vi "Actor Core.vi"(8 "error in":cluster{"状态":bool, "代码":i32, "源":string} caption="错误输入", 11 "我的应用程序":refnum<class "多对一.lvclass">) -> (0 "error out":cluster{"状态":bool, "代码":i32, "源":string} caption="错误输出", 3 "操作者输出":refnum<class "Actor.lvclass">)   [LabVIEW 2015, in "多对一.lvlib" / "多对一.lvclass"]
doc: "Actor Core.vi包含操作者的主要消息处理循环。操作者通常位于该循环中，在各种消息到达时对消息进行处理。如Do.vi消息返回任何错误，该循环将停止运行，错误代码43将被作为“无错误停止”的标准信号发送给调用方。如需更改上述行为，可在子孙类的Handle Error.vi中对该部分逻辑进行重写。"
uses:
  <vilib>/ActorFramework/Actor/Actor.lvclass
  <vilib>/ActorFramework/Stop Msg/Stop Msg.lvclass
panel:
  in  "停止信号":bool
  out "事件记录":string
  in  "停止":bool
  in  "至客户端的消息":bool
  in  "至硬件的消息":bool
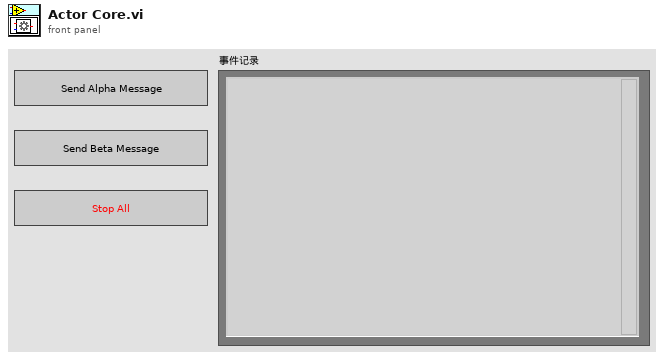
[diagram p1: front panel]
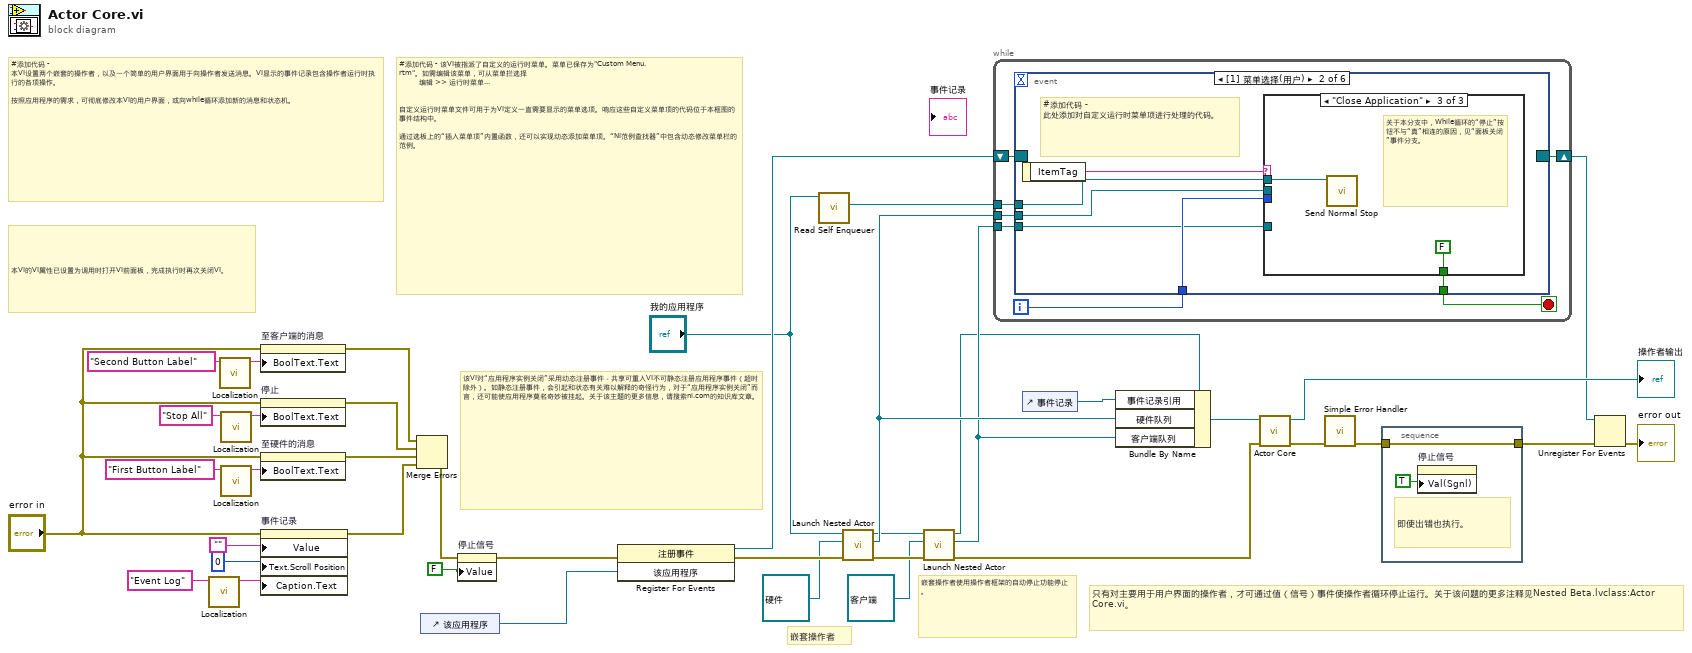
[diagram p0: block diagram]
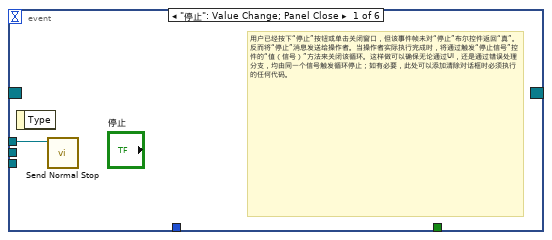
[diagram p2: hidden frame]
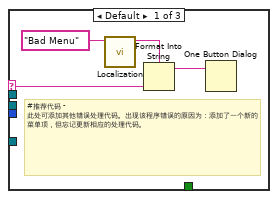
[diagram p3: hidden frame]
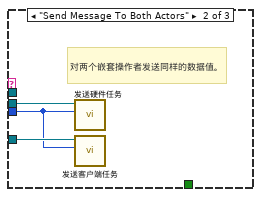
[diagram p4: hidden frame]
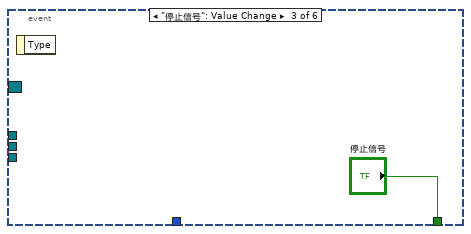
[diagram p5: hidden frame]
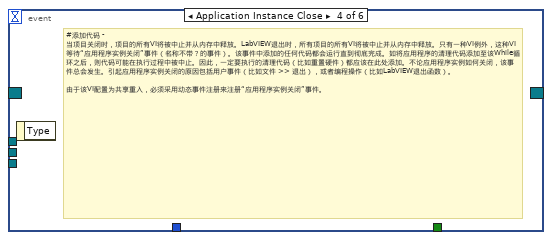
[diagram p6: hidden frame]
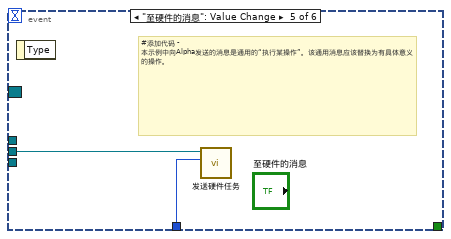
[diagram p7: hidden frame]
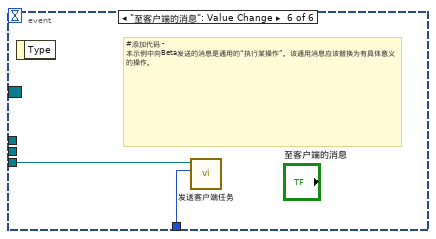
[diagram p8: hidden frame]
diagram:
  # "嵌套操作者"
  # "嵌套操作者使用操作者框架的自动停止功能停止。"
  # "#添加代码 - 该VI被指派了自定义的运行时菜单。菜单已保存为\"Custom Menu.rtm\"。如需编辑该菜单，可从菜单拦选择\n          编辑 >> 运行时菜单...\n\n\n自定义运行时菜单文件可用于为VI定义一直需要显示的菜单选项。响应这些自定义菜单项的代码位于本框图的事件结构中。\n\n通过选板上的“插入菜单项”内置函数，还可以实现动态添加菜单项。“NI范例查找器”中包含动态修改菜单栏的范例。"
  # "该VI对“应用程序实例关闭”采用动态注册事件－共享可重入VI不可静态注册应用程序事件（超时除外）。如静态注册事件，会引起和状态有关难以解释的奇怪行为，对于“应用程序实例关闭”而言，还可能使应用程序莫名奇妙被挂起。关于该主题的更多信息，请搜索ni.com的知识库文章。"
  # "本VI的VI属性已设置为调用时打开VI前面板，完成执行时再次关闭VI。"
  # "只有对主要用于用户界面的操作者，才可通过值（信号）事件使操作者循环停止运行。关于该问题的更多注释见Nested Beta.lvclass:Actor Core.vi。"
  # "#添加代码 - 本VI设置两个嵌套的操作者，以及一个简单的用户界面用于向操作者发送消息。VI显示的事件记录包含操作者运行时执行的各项操作。\n\n按照应用程序的需求，可彻底修改本VI的用户界面，或向while循环添加新的消息和状态机。"
  n1 = call "Localization.vi"("未本地化"="Event Log" ("Unlocalized")) -> ("本地化"=w26:string)  [unwired: 10 in]
  n2 = call "Localization.vi"("未本地化"="Second Button Label" ("Unlocalized")) -> ("本地化"=w20:string)  [unwired: 10 in]
  n3 = call "Localization.vi"("未本地化"="Stop All" ("Unlocalized")) -> ("本地化"=w22:string)  [unwired: 10 in]
  n4 = call "Localization.vi"("未本地化"="First Button Label" ("Unlocalized")) -> ("本地化"=w24:string)  [unwired: 10 in]
  n5 = property on="至客户端的消息" class="Bool"(error in="error in", "BoolText.Text"=w20) -> (error out=w19:errorcluster)  [unwired: 1 in, 1 out]
  n6 = property on="停止" class="Bool"(error in="error in", "BoolText.Text"=w22) -> (error out=w18:errorcluster)  [unwired: 1 in, 1 out]
  n7 = property on="至硬件的消息" class="Bool"(error in="error in", "BoolText.Text"=w24) -> (error out=w17:errorcluster)  [unwired: 1 in, 1 out]
  n8 = property on="事件记录" class="Str"(error in="error in", "Value"="" ("Empty String Constant"), "Text.Scroll Position"=u32 0, "Caption.Text"=w26) -> (error out=w16:errorcluster)  [unwired: 1 in, 1 out]
  n9 = Merge Errors(w19, w18, w17, w16) -> (w15:errorcluster)
  n10 = control-ref of="该应用程序"() -> (w6:refnum<vi>)
  n11 = property on="停止信号" class="Bool (严格)"(error in=w15, "Value"=FALSE ("stop")) -> (error out=w8:errorcluster)  [unwired: 1 in, 1 out]
  n12 = register-events(error in=w8, w6) -> (reference out=w12:refnum<event-registration>, error out=w7:errorcluster)  [unwired: 1 in]
  n13 = call <vilib>:"Read Self Enqueuer.vi"("Actor"="我的应用程序") -> ("Self Enqueuer"=w34:refnum<class "Message Enqueuer.lvclass">)  [unwired: 10 in]
  n14 = call <vilib>:"Launch Nested Actor.vi"("error in (no error)"=w7, "Nested Actor"=refnum<class "硬件.lvclass"> refnum ("Alpha.lvclass"), "Caller Actor in"="我的应用程序") -> ("error out"=w38:errorcluster, "Nested Actor's Enqueuer"=w33:refnum<class "Message Enqueuer.lvclass">, "Caller Actor out"=w4:refnum<class "多对一.lvclass">)  [unwired: 6 in]
  n15 = call <vilib>:"Launch Nested Actor.vi"("error in (no error)"=w38, "Nested Actor"=refnum<class "客户端.lvclass"> refnum ("Beta.lvclass"), "Caller Actor in"=w4) -> ("error out"=w37:errorcluster, "Nested Actor's Enqueuer"=w32:refnum<class "Message Enqueuer.lvclass">, "Caller Actor out"=w1:refnum<class "多对一.lvclass">)  [unwired: 6 in]
  n16 = while {
    tunnel: w34 -> [w46]
    tunnel: w33 -> [w45]
    tunnel: w32 -> [w44]
    shift-right: [w40] -> w11
    shift-left: w12 -> [w41]
    i -> [w42]
    stop <- w43 stop-if-true
    n17 = event shown="[1] 菜单选择(用户)" {
      selector: w41 -> [_ _ _ _ _ _]
      dyn-events: [_ _ _ _ _ _] -> w40
      timeout: _ -> [_ _ _ _ _ _]
      tunnel: w46 -> [w47 w49 _ _ _ _]
      tunnel: w45 -> [_ w52 _ _ w65 _]
      tunnel: w44 -> [_ w50 _ _ _ w67]
      tunnel: [_ w48 "停止信号" _ _ _] -> w43
      tunnel: w42 -> [_ w51 _ _ w64 w66]
      event "停止": Value Change; Panel Close {
        # "用户已经按下“停止”按钮或单击关闭窗口，但该事件帧未对“停止”布尔控件返回“真”。反而将“停止”消息发送给操作者。当操作者实际执行完成时，将通过触发“停止信号”控件的“值（信号）”方法来关闭该循环。这样做可以确保无论通过UI，还是通过错误处理分支，均由同一个信号触发循环停止；如有必要，此处可以添加清除对话框时必须执行的任何代码。"
        n18 = event-data() -> ()  [unwired: 1 in, 1 out]
        n19 = call <vilib>:"Send Normal Stop.vi"("Message Enqueuer"=w47) -> ()  [unwired: 10 in, 1 out]
      }
      event Menu Selection (User) {
        # "#添加代码 - 此处添加对自定义运行时菜单项进行处理的代码。"
        n20 = event-data() -> ("ItemTag"=w53:string)  [unwired: 1 in]
        n21 = case shown="\"Close Application\"" w53 {
          selector: w53 -> [w55 _ _]
          tunnel: w52 -> [_ w60 _]
          tunnel: w51 -> [_ w58 _]
          tunnel: w50 -> [_ w59 _]
          tunnel: w49 -> [_ _ w62]
          tunnel: [_ _ FALSE] -> w48
          frame Default {
            # "#推荐代码 - 此处可添加其他错误处理代码。出现该程序错误的原因为：添加了一个新的菜单项，但忘记更新相应的处理代码。"
            n22 = call "Localization.vi"("未本地化"="Bad Menu" ("Unlocalized")) -> ("本地化"=w56:string)  [unwired: 10 in]
            n23 = Format Into String(format string=w56, w55) -> (resulting string=w54:string)  [unwired: 2 in, 1 out]
            n24 = One Button Dialog(message=w54) -> ()  [unwired: 1 in, 1 out]
          }
          frame "Send Message To Both Actors" {
            # "对两个嵌套操作者发送同样的数据值。"
            n25 = call "发送硬件任务.vi"("数据"=w58, "消息待入队列"=w60) -> ()  [unwired: 9 in, 1 out]
            n26 = call "发送客户端任务.vi"("数据"=w58, "消息待入队列"=w59) -> ()  [unwired: 9 in, 1 out]
          }
          frame "Close Application" {
            # "关于本分支中，While循环的“停止”按钮不与“真”相连的原因，见“面板关闭”事件分支。"
            n27 = call <vilib>:"Send Normal Stop.vi"("Message Enqueuer"=w62) -> ()  [unwired: 10 in, 1 out]
          }
        }
      }
      event "停止信号": Value Change {
        n28 = event-data() -> ()  [unwired: 1 in, 1 out]
      }
      event Application Instance Close {
        # "#添加代码 - 当项目关闭时，项目的所有VI将被中止并从内存中释放。LabVIEW退出时，所有项目的所有VI将被中止并从内存中释放。只有一种VI例外，这种VI等待“应用程序实例关闭”事件（名称不带？的事件）。该事件中添加的任何代码都会运行直到彻底完成。如将应用程序的清理代码添加至该While循环之后，则代码可能在执行过程中被中止。因此，一定要执行的清理代码（比如重置硬件）都应该在此处添加。不论应用程序实例如何关闭，该事件总会发生。引起应用程序实例关闭的原因包括用户事件（比如文件 >> 退出），或者编程操作（比如LabVIEW退出函数）。\n\n由于该VI配置为共享重入，必须采用动态事件注册来注册“应用程序实例关闭”事件。"
        n29 = event-data() -> ()  [unwired: 1 in, 1 out]
      }
      event "至硬件的消息": Value Change {
        # "#添加代码 - 本示例中向Alpha发送的消息是通用的“执行某操作”。该通用消息应该替换为有具体意义的操作。"
        n30 = event-data() -> ()  [unwired: 1 in, 1 out]
        n31 = call "发送硬件任务.vi"("数据"=w64, "消息待入队列"=w65) -> ()  [unwired: 9 in, 1 out]
      }
      event "至客户端的消息": Value Change {
        # "#添加代码 - 本示例中向Beta发送的消息是通用的“执行某操作”。该通用消息应该替换为有具体意义的操作。"
        n32 = event-data() -> ()  [unwired: 1 in, 1 out]
        n33 = call "发送客户端任务.vi"("数据"=w66, "消息待入队列"=w67) -> ()  [unwired: 9 in, 1 out]
      }
    }
  }
  n34 = control-ref of="事件记录"() -> (w35:refnum<vi>)
  n35 = Bundle By Name(cluster=w1, "事件记录引用"=w35, "硬件队列"=w33, "客户端队列"=w32) -> (w36:refnum<class "多对一.lvclass">)
  n36 = call-parent "Actor Core.vi"("error in"=w37, "Actor in"=w36) -> ("error out"=w14:errorcluster, "Actor out"=→"操作者输出":refnum<class "Actor.lvclass">)  [unwired: 8 in]
  n37 = call <vilib>:"Simple Error Handler.vi"("error in (no error)"=w14) -> ("error out"=w13:errorcluster)  [unwired: 4 in, 4 out]
  n38 = stacked-sequence {
    tunnel: [w68] -> w10
    tunnel: w13 -> [w68]
    frame #0 {
      # "即使出错也执行。"
      n39 = property on="停止信号" class="Bool (严格)"("Val(Sgnl)"=TRUE ("stop")) -> ()  [unwired: 2 in, 2 out]
    }
  }
  n40 = Unregister For Events(event registration refnum=w11, error in=w10) -> (error out=→"error out":errorcluster)
